vi "CreateUserEvent.vi"() -> (0 "error out":errorcluster, 3 "User Event out":refnum<user-event>)   [LabVIEW 2018]
doc: "Collegamento di comunicazione per gli userevent"
uses:
  Desktop/StateMachineTest/2/Messages.ctl
  MessageCluster.ctl
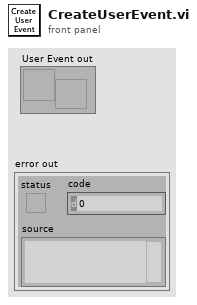
[diagram p1: front panel]
types:
  T1 = typedef "MessageCluster.ctl" = cluster{"Message":string, "Temp":i32, "Stato":enum16{"On", "Off", "Preparation", "WaitTimer", "Ready"}}
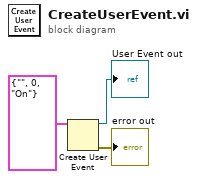
[diagram p0: block diagram]
diagram:
  n1 = Create User Event(user event datatype=T1 {"Message"="", "Temp"=0, "Stato"=enum."On"} ("Message Cluster")) -> (user event=→"User Event out":refnum<user-event>, error out=→"error out":errorcluster)  [unwired: 1 in]
